vi "Victor Linearize.vi"(10 "Goal Speed":dbl) -> (2 "Output":dbl)   [LabVIEW 2013]
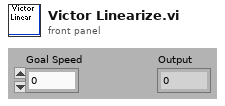
[diagram p1: front panel]
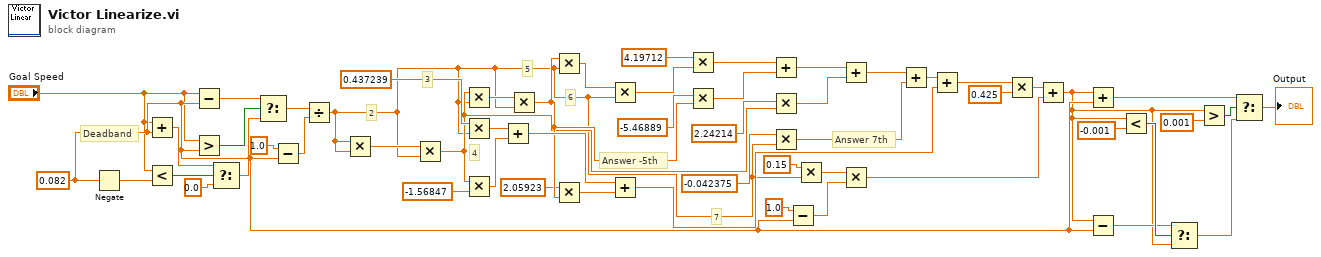
[diagram p0: block diagram]
diagram:
  w9 = 0.082
  # "Answer 7th"
  # "Answer -5th"
  # "7"
  # "6"
  # "5"
  # "4"
  # "3"
  # "2"
  # "Deadband"
  n1 = Negate(x=w9) -> (-x=w52:dbl)
  n2 = Add(x="Goal Speed", y=w9) -> (x+y=w6:dbl)
  n3 = Less?(x="Goal Speed", y=w52) -> (x < y?=w53:bool)
  n4 = Subtract(x="Goal Speed", y=w9) -> (x-y=w50:dbl)
  n5 = Greater?(x="Goal Speed", y=w9) -> (0:w55:bool)
  n6 = Select(t=w6, s=w53, f=0.0) -> (s? t:f=w54:dbl)
  n7 = Select(t=w50, s=w55, f=w54) -> (s? t:f=w49:dbl)
  n8 = Subtract(x=1.0, y=w9) -> (x-y=w47:dbl)
  n9 = Divide(x=w49, y=w47) -> (x/y=w20:dbl)
  n10 = Multiply(x=w20, y=w20) -> (x*y=w46:dbl)
  n11 = Multiply(x=w46, y=w20) -> (x*y=w32:dbl)
  n12 = Multiply(x=w32, y=w20) -> (x*y=w45:dbl)
  n13 = Multiply(x=0.437239, y=w20) -> (x*y=w41:dbl)
  n14 = Multiply(x=w32, y=-1.56847) -> (x*y=w40:dbl)
  n15 = Add(x=w41, y=w40) -> (x+y=w38:dbl)
  n16 = Multiply(x=w45, y=w20) -> (x*y=w34:dbl)
  n17 = Multiply(x=w34, y=w20) -> (x*y=w44:dbl)
  n18 = Multiply(x=2.05923, y=w34) -> (x*y=w39:dbl)
  n19 = Multiply(x=w44, y=w20) -> (x*y=w36:dbl)
  n20 = Add(x=w38, y=w39) -> (x+y=w24:dbl)
  n21 = Multiply(x=4.19712, y=w36) -> (x*y=w30:dbl)
  n22 = Multiply(x=-5.46889, y=w34) -> (x*y=w29:dbl)
  n23 = Add(x=w30, y=w29) -> (x+y=w27:dbl)
  n24 = Multiply(x=2.24214, y=w32) -> (x*y=w28:dbl)
  n25 = Multiply(x=-0.042375, y=w20) -> (x*y=w26:dbl)
  n26 = Subtract(x=1.0, y=w9) -> (x-y=w18:dbl)
  n27 = Multiply(x=0.15, y=w20) -> (x*y=w17:dbl)
  n28 = Add(x=w27, y=w28) -> (x+y=w37:dbl)
  n29 = Multiply(x=w17, y=w18) -> (x*y=w16:dbl)
  n30 = Add(x=w37, y=w26) -> (x+y=w25:dbl)
  n31 = Add(x=w25, y=w24) -> (x+y=w23:dbl)
  n32 = Multiply(x=w23, y=0.425) -> (x*y=w15:dbl)
  n33 = Add(x=w15, y=w16) -> (x+y=w7:dbl)
  n34 = Add(x=w7, y=w9) -> (x+y=w12:dbl)
  n35 = Subtract(x=w7, y=w9) -> (x-y=w8:dbl)
  n36 = Less?(x=w7, y=-0.001) -> (x < y?=w10:bool)
  n37 = Select(t=w8, s=w10, f=w7) -> (s? t:f=w4:dbl)
  n38 = Greater?(x=w7, y=0.001) -> (0:w13:bool)
  n39 = Select(t=w12, s=w13, f=w4) -> (s? t:f=→"Output":dbl)
